vi "1 Tap 24-Bit RGB.vi"() -> (0 "Pixels":cluster{"Pixel 0":u32})   [LabVIEW 2015]
uses:
  <vilib>/eio/EIONode/EIONode.xnode
  <vilib>/rvi/eio/common/nirviEmuTemplateMethod_errors.vi
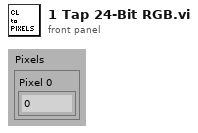
[diagram p1: front panel]
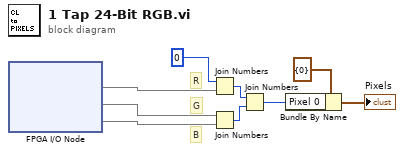
[diagram p0: block diagram]
diagram:
  # "B"
  # "G"
  # "R"
  n1 = xnode "FPGA I/O Node"() -> ("CL Port A"=w7, "CL Port B"=w8, "CL Port C"=w9)  [unwired: 3 in, 3 out]
  n2 = Join Numbers(hi=u8 0, lo=w7) -> ((hi.lo)=w4:u16)
  n3 = Join Numbers(hi=w8, lo=w9) -> ((hi.lo)=w5:u32)
  n4 = Join Numbers(hi=w4, lo=w5) -> ((hi.lo)=w3:u64)
  n5 = Bundle By Name(cluster=cluster{"Pixel 0":u32} {"Pixel 0"=0} ("Data"), "Pixel 0"=w3) -> (→"Pixels":cluster{"Pixel 0":u32})
